vi "setShifterName.vi"(8 "error in (no error)":errorcluster, 10 "Shifter Name":string, 11 "Shift in":refnum<class "Shift.lvclass">) -> (0 "error out":errorcluster, 3 "Shift out":refnum<class "Shift.lvclass">)   [LabVIEW 2013, in "Shift.lvclass"]
uses:
  Shift.lvclass
  Shift.lvclass/Shift.ctl
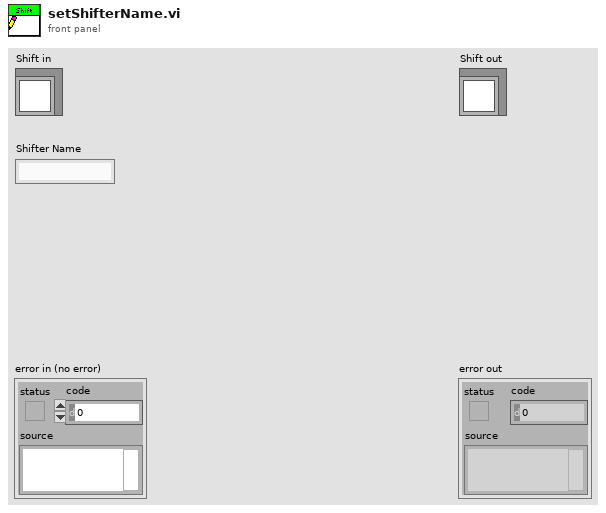
[diagram p1: front panel]
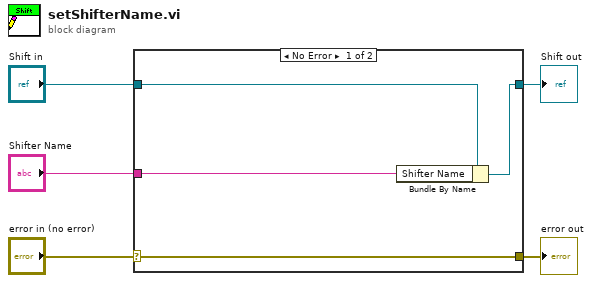
[diagram p0: block diagram]
diagram:
  n1 = case shown="No Error" "error in (no error)" {
    selector: "error in (no error)" -> [w9 w10]
    tunnel: [w9 w10] -> w4
    tunnel: [w7 w11] -> w2
    tunnel: "Shift in" -> [w8 w11]
    tunnel: "Shifter Name" -> [w6 _]
    frame No Error {
      n2 = Bundle By Name(cluster=w8, "Shifter Name"=w6) -> (w7:refnum<class "Shift.lvclass">)
    }
    frame Error {
    }
  }
  "error out" <- w4
  "Shift out" <- w2
